vi "AvgTempFlowsLabels.vi"(6 "LabVIEW Web Service Request":refnum<class "Web Request.lvclass">) -> (0 "AvgTempsLabels":T1(array[cluster]), 1 "TempData":bool=TRUE, 2 "FuelData":bool=TRUE, 3 "AvgFuelsLabels":T1(array[cluster]))   [LabVIEW 2017]
uses:
  <vilib>/wsapi/Web Request.lvclass
panel:
  # "Use the Web Service Request input terminal to call the VIs on the Web Services palette. Do not remove it from the connector pane unless you don't need access to the palette."
  # "Each additional control wired to the connector pane will be available as an input in the URL. To include an indicator in terminal-mode output (the default setting), it must also be wired to the connector pane."
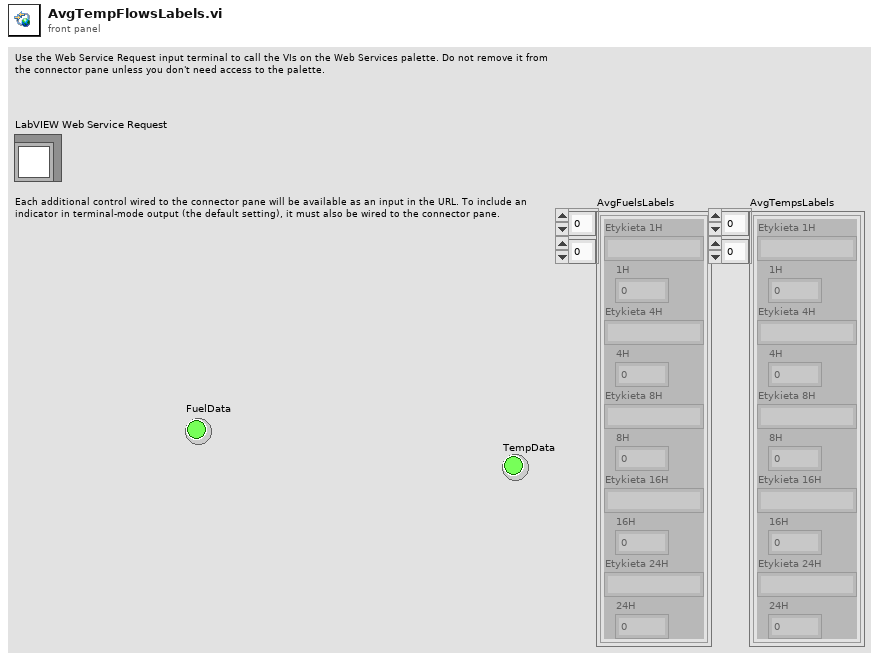
[diagram p1: front panel]
types:
  T1 = cluster{"Etykieta 1H":string, "1H":dbl, "Etykieta 4H":string, "4H":dbl, "Etykieta 8H":string, "8H":dbl, "Etykieta 16H":string, "16H":dbl, "Etykieta 24H":string, "24H":dbl}[][]
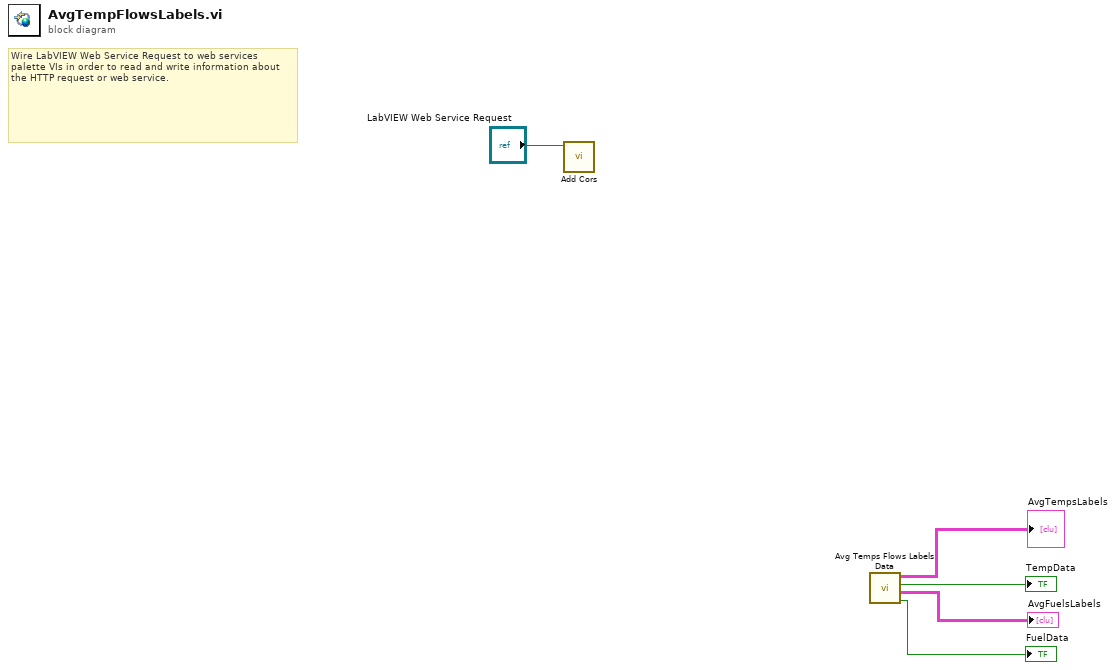
[diagram p0: block diagram]
diagram:
  # "Wire LabVIEW Web Service Request to web services palette VIs in order to read and write information about the HTTP request or web service."
  n1 = call "Add Cors.vi"("Web Request in"="LabVIEW Web Service Request") -> ()  [unwired: 10 in, 1 out]
  n2 = call "Avg Temps Flows Labels Data.vi"() -> ("FuelData"=→"FuelData":bool, "AvgFuelsLabels"=→"AvgFuelsLabels":T1, "TempData"=→"TempData":bool, "AvgTempsLabels"=→"AvgTempsLabels":T1)  [unwired: 8 in]
